vi "Send PEM Command (No time).vi"(8 "error in (no error)":errorcluster, 10 "query string":string, 11 "VISA resource name":refnum<visa-resource-name>="COM1") -> (0 "error out":errorcluster, 1 "read buffer":string, 2 "read buffer 2":string, 3 "VISA resource name out":refnum<visa-resource-name>)   [LabVIEW 2017]
panel:
  in  "Bytes Count":u32=1024
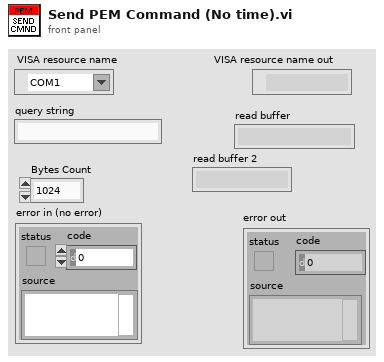
[diagram p1: front panel]
types:
  T1 = typedef "Semaphore RefNum" = refnum<k1>
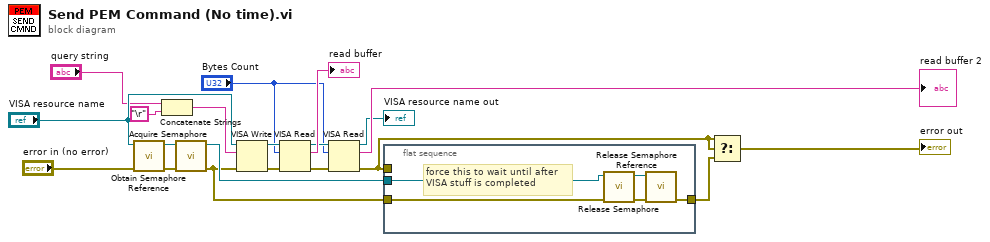
[diagram p0: block diagram]
diagram:
  n1 = call <vilib>:"Obtain Semaphore Reference.vi"("error in (no error)"="error in (no error)", "name (unnamed)"="VISA resource name") -> ("error out"=w17:errorcluster, "semaphore"=w18:T1)  [unwired: 1 in, 3 out]
  n2 = Concatenate Strings("query string", "\r") -> (w4:string)
  n3 = call <vilib>:"Acquire Semaphore.vi"("error in (no error)"=w17, "semaphore"=w18) -> ("error out"=w12:errorcluster, "semaphore out"=w15:T1)  [unwired: 1 in, 3 out]
  n4 = VISA Write(VISA resource name="VISA resource name", write buffer=w4, error in (no error)=w12) -> (VISA resource name out=w20:refnum<visa-resource-name>, error out=w19:errorcluster)  [unwired: 1 out]
  n5 = VISA Read(VISA resource name=w20, byte count="Bytes Count", error in (no error)=w19) -> (VISA resource name out=w10:refnum<visa-resource-name>, read buffer=→"read buffer":string, error out=w9:errorcluster)  [unwired: 1 out]
  n6 = VISA Read(VISA resource name=w10, byte count="Bytes Count", error in (no error)=w9) -> (VISA resource name out=→"VISA resource name out":refnum<visa-resource-name>, read buffer=→"read buffer 2":string, error out=w3:errorcluster)  [unwired: 1 out]
  n7 = flat-sequence {
    tunnel: w15 -> [w25]
    tunnel: [w22] -> w13
    tunnel: w12 -> [w21]
    tunnel: w3 -> [_]
    frame #0 {
      # "force this to wait until after \nVISA stuff is completed"
      n8 = call <vilib>:"Release Semaphore.vi"("error in (no error)"=w21, "semaphore"=w25) -> ("error out"=w23:errorcluster, "semaphore out"=w24:T1)  [unwired: 4 out]
      n9 = call <vilib>:"Release Semaphore Reference.vi"("error in (no error)"=w23, "semaphore"=w24) -> ("error out"=w22:errorcluster)  [unwired: 9 out]
    }
  }
  n10 = Select(t=w3, s=w3, f=w13) -> (s? t:f=→"error out":errorcluster)
